vi "Handle Last Ack Core.vi"(4 "error in (no error)":errorcluster, 6 "Last Ack":refnum<class "Last Ack.lvclass">, 7 "PVClient-Example in":refnum<class "PVClient-Example.lvclass">) -> (0 "error out":errorcluster, 3 "PVClient-Example out":refnum<class "PVClient-Example.lvclass">)   [LabVIEW 2014, in "PVClient-Example.lvlib" / "PVClient-Example.lvclass"]
doc: "(<B>Filename</B>: Actor Framework.lvlib:Actor.lvclass:Handle Last Ack Core.vi)\n\nDefines how the caller actor responds to the Last Ack message from a nested actor. The Last Ack message is the final message a nested actor sends to its caller before it shuts down. The message contains information about the final state of the nested actor.\n\nBy default, this method does nothing except return any error the nested actor sent. A descendant class may override this method to define behavior."
uses:
  PVClient-Example.lvclass
  <vilib>/ActorFramework/LastAck/Last Ack.lvclass
  PVClient-Example.lvclass/PVClient-Example.ctl
  CSPP_Core/Actors/CS++BaseActor/CS++BaseActor.lvclass
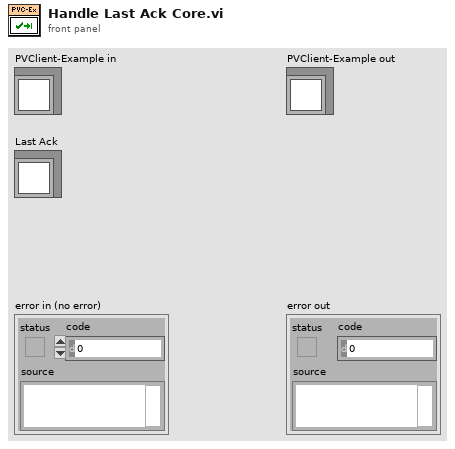
[diagram p1: front panel]
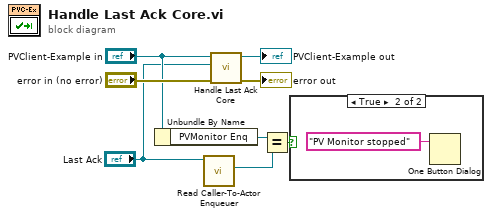
[diagram p0: block diagram]
diagram:
  n1 = Unbundle By Name("PVClient-Example in") -> ("PVMonitor Enq"=w4:refnum<class "Message Enqueuer.lvclass">)
  n2 = call <vilib>:"Read Caller-To-Actor Enqueuer.vi"("Last Ack"="Last Ack") -> ("Caller-to-Actor Enqueuer"=w3:refnum<class "Message Enqueuer.lvclass">)  [unwired: 10 in]
  n3 = call-parent "Handle Last Ack Core.vi"("error in (no error)"="error in (no error)", "Last Ack"="Last Ack", "Actor in"="PVClient-Example in") -> ("error out"=→"error out":errorcluster, "Actor out"=→"PVClient-Example out":refnum<class "PVClient-Example.lvclass">)  [unwired: 3 in]
  n4 = Equal?(x=w4, y=w3) -> (x = y?=w1:bool)
  n5 = case shown="True" w1 {
    frame False {
    }
    frame True {
      n6 = One Button Dialog(message="PV Monitor stopped") -> ()  [unwired: 1 in, 1 out]
    }
  }
